vi "Config - access SUM report - REPORT.vi"(5 ".ini Controller":enum16{"Read", "Write"}(ring), 6 "End Time":timestamp, 7 "Start Time":timestamp, 8 "error in":errorcluster, 9 "RVHR Cluster In":T1, 10 "Cluster in":T7 {"Settings Cluster"."Image Frequency" items=["2", "3", "5"]; "Settings Cluster"."Device Resolution" items=["0.1 µm", "1 µm", "10 µm"]; "Settings Cluster"."Distance Format" items=["kilometres", "miles & chains", "metres", "stations", "miles"]; "Settings Cluster"."Sampling Distance" items=["1mm", "2mm"]}, 11 "Config File Ref":T14=refnum) -> (0 "error out":errorcluster, 1 "Dates-Times":T6, 2 "Cluster out":T7 {"Settings Cluster"."Image Frequency" items=["2", "3", "5"]; "Settings Cluster"."Device Resolution" items=["0.1 µm", "1 µm", "10 µm"]; "Settings Cluster"."Distance Format" items=["kilometres", "miles & chains", "metres", "stations", "miles"]; "Settings Cluster"."Sampling Distance" items=["1mm", "2mm"]}, 3 "refnum out":T14)   [LabVIEW 2023]
doc: "This subVI reads/writes initial config data from a .ini file to define the test settings."
uses:
  Controls/File Information CLuster.ctl
  Controls/Run Description.ctl
  Controls/Run information (YRCA).ctl
  Controls/System information (YRCA - Truncate).ctl
  Controls/Sum File Cluster (RCA).ctl
  Controls/Sampling DIstance.ctl
  <vilib>/Utility/config.llb/Config Data RefNum.ctl
  <vilib>/Utility/config.llb/NI_LVConfig.lvlib
  Controls/SUM Cluster.ctl
  Controls/Test Cluster.ctl
  Controls/Distance Units.ctl
  Controls/Settings Cluster.ctl
  Controls/Device_Type.ctl
  Controls/Device_Resolution.ctl
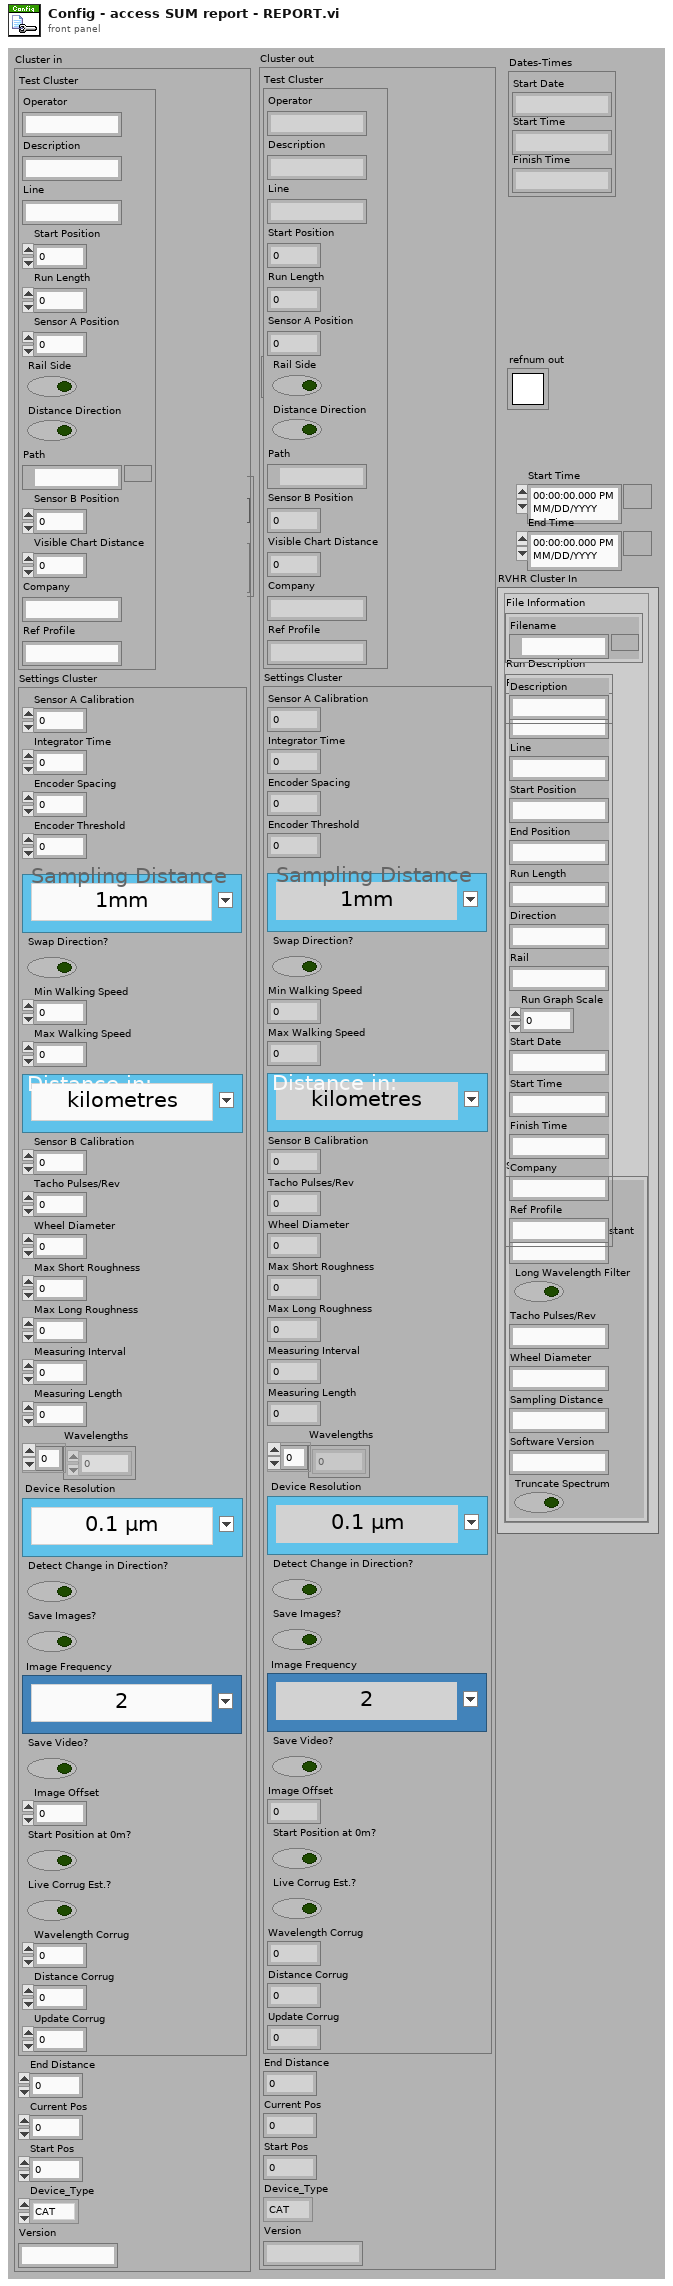
[diagram p1: front panel]
types:
  T1 = typedef "Sum File Cluster (RCA).ctl" = cluster{"File Information":T2, "Run Description":T3, "Run Information":T4, "System Information":T5}
  T2 = typedef "File Information CLuster.ctl" = cluster{"Filename":path}
  T3 = typedef "Run Description.ctl" = cluster{"Description":string}
  T4 = typedef "Run information (YRCA).ctl" = cluster{"Operator":string, "Line":string, "Start Position":string, "End Position":string, "Run Length":string, "Direction":string, "Rail":string, "Run Graph Scale":u16, "Start Date":string, "Start Time":string, "Finish Time":string, "Company":string, "Ref Profile":string}
  T5 = typedef "System information (YRCA - Truncate).ctl" = cluster{"Sensor Calibration":string, "Integrator Time Constant":string, "Long Wavelength Filter":bool, "Tacho Pulses/Rev":string, "Wheel Diameter":string, "Sampling Distance":string, "Software Version":string, "Truncate Spectrum":bool}
  T6 = cluster{"Start Date":string, "Start Time":string, "Finish Time":string}
  T7 = typedef "SUM Cluster.ctl" = cluster{"Test Cluster":T8, "Settings Cluster":T9, "End Distance":dbl, "Current Pos":dbl, "Start Pos":dbl, "Device_Type":T13, "Version":string}
  T8 = typedef "Test Cluster.ctl" = cluster{"Operator":string, "Description":string, "Line":string, "Start Position":dbl, "Run Length":dbl, "Sensor A Position":dbl, "Rail Side":bool, "Distance Direction":bool, "Path":path, "Sensor B Position":dbl, "Visible Chart Distance":dbl, "Company":string, "Ref Profile":string}
  T9 = typedef "Settings Cluster.ctl" = cluster{"Sensor A Calibration":dbl, "Integrator Time":dbl, "Encoder Spacing":dbl, "Encoder Threshold":dbl, "Sampling Distance":T10, "Swap Direction?":bool, "Min Walking Speed":dbl, "Max Walking Speed":dbl, "Distance Format":T11, "Sensor B Calibration":dbl, "Tacho Pulses/Rev":dbl, "Wheel Diameter":dbl, "Max Short Roughness":dbl, "Max Long Roughness":dbl, "Measuring Interval":dbl, "Measuring Length":dbl, "Wavelengths":dbl[], "Device Resolution":T12, "Detect Change in Direction?":bool, "Save Images?":bool, "Image Frequency":T10, "Save Video?":bool, "Image Offset":dbl, "Start Position at 0m?":bool, "Live Corrug Est.?":bool, "Wavelength Corrug":u8, "Distance Corrug":u8, "Update Corrug":u8}
  T10 = typedef "Sampling DIstance.ctl" = u16
  T11 = typedef "Distance Units.ctl" = u16
  T12 = typedef "Device_Resolution.ctl" = u16
  T13 = typedef "Device_Type.ctl" = enum16{"CAT", "Bi-CAT", "YRCA", "RCA", "RV-HR", "TV-HR"}
  T14 = typedef "NI_LVConfig.lvlib/Config Data RefNum.ctl" = refnum<k1>
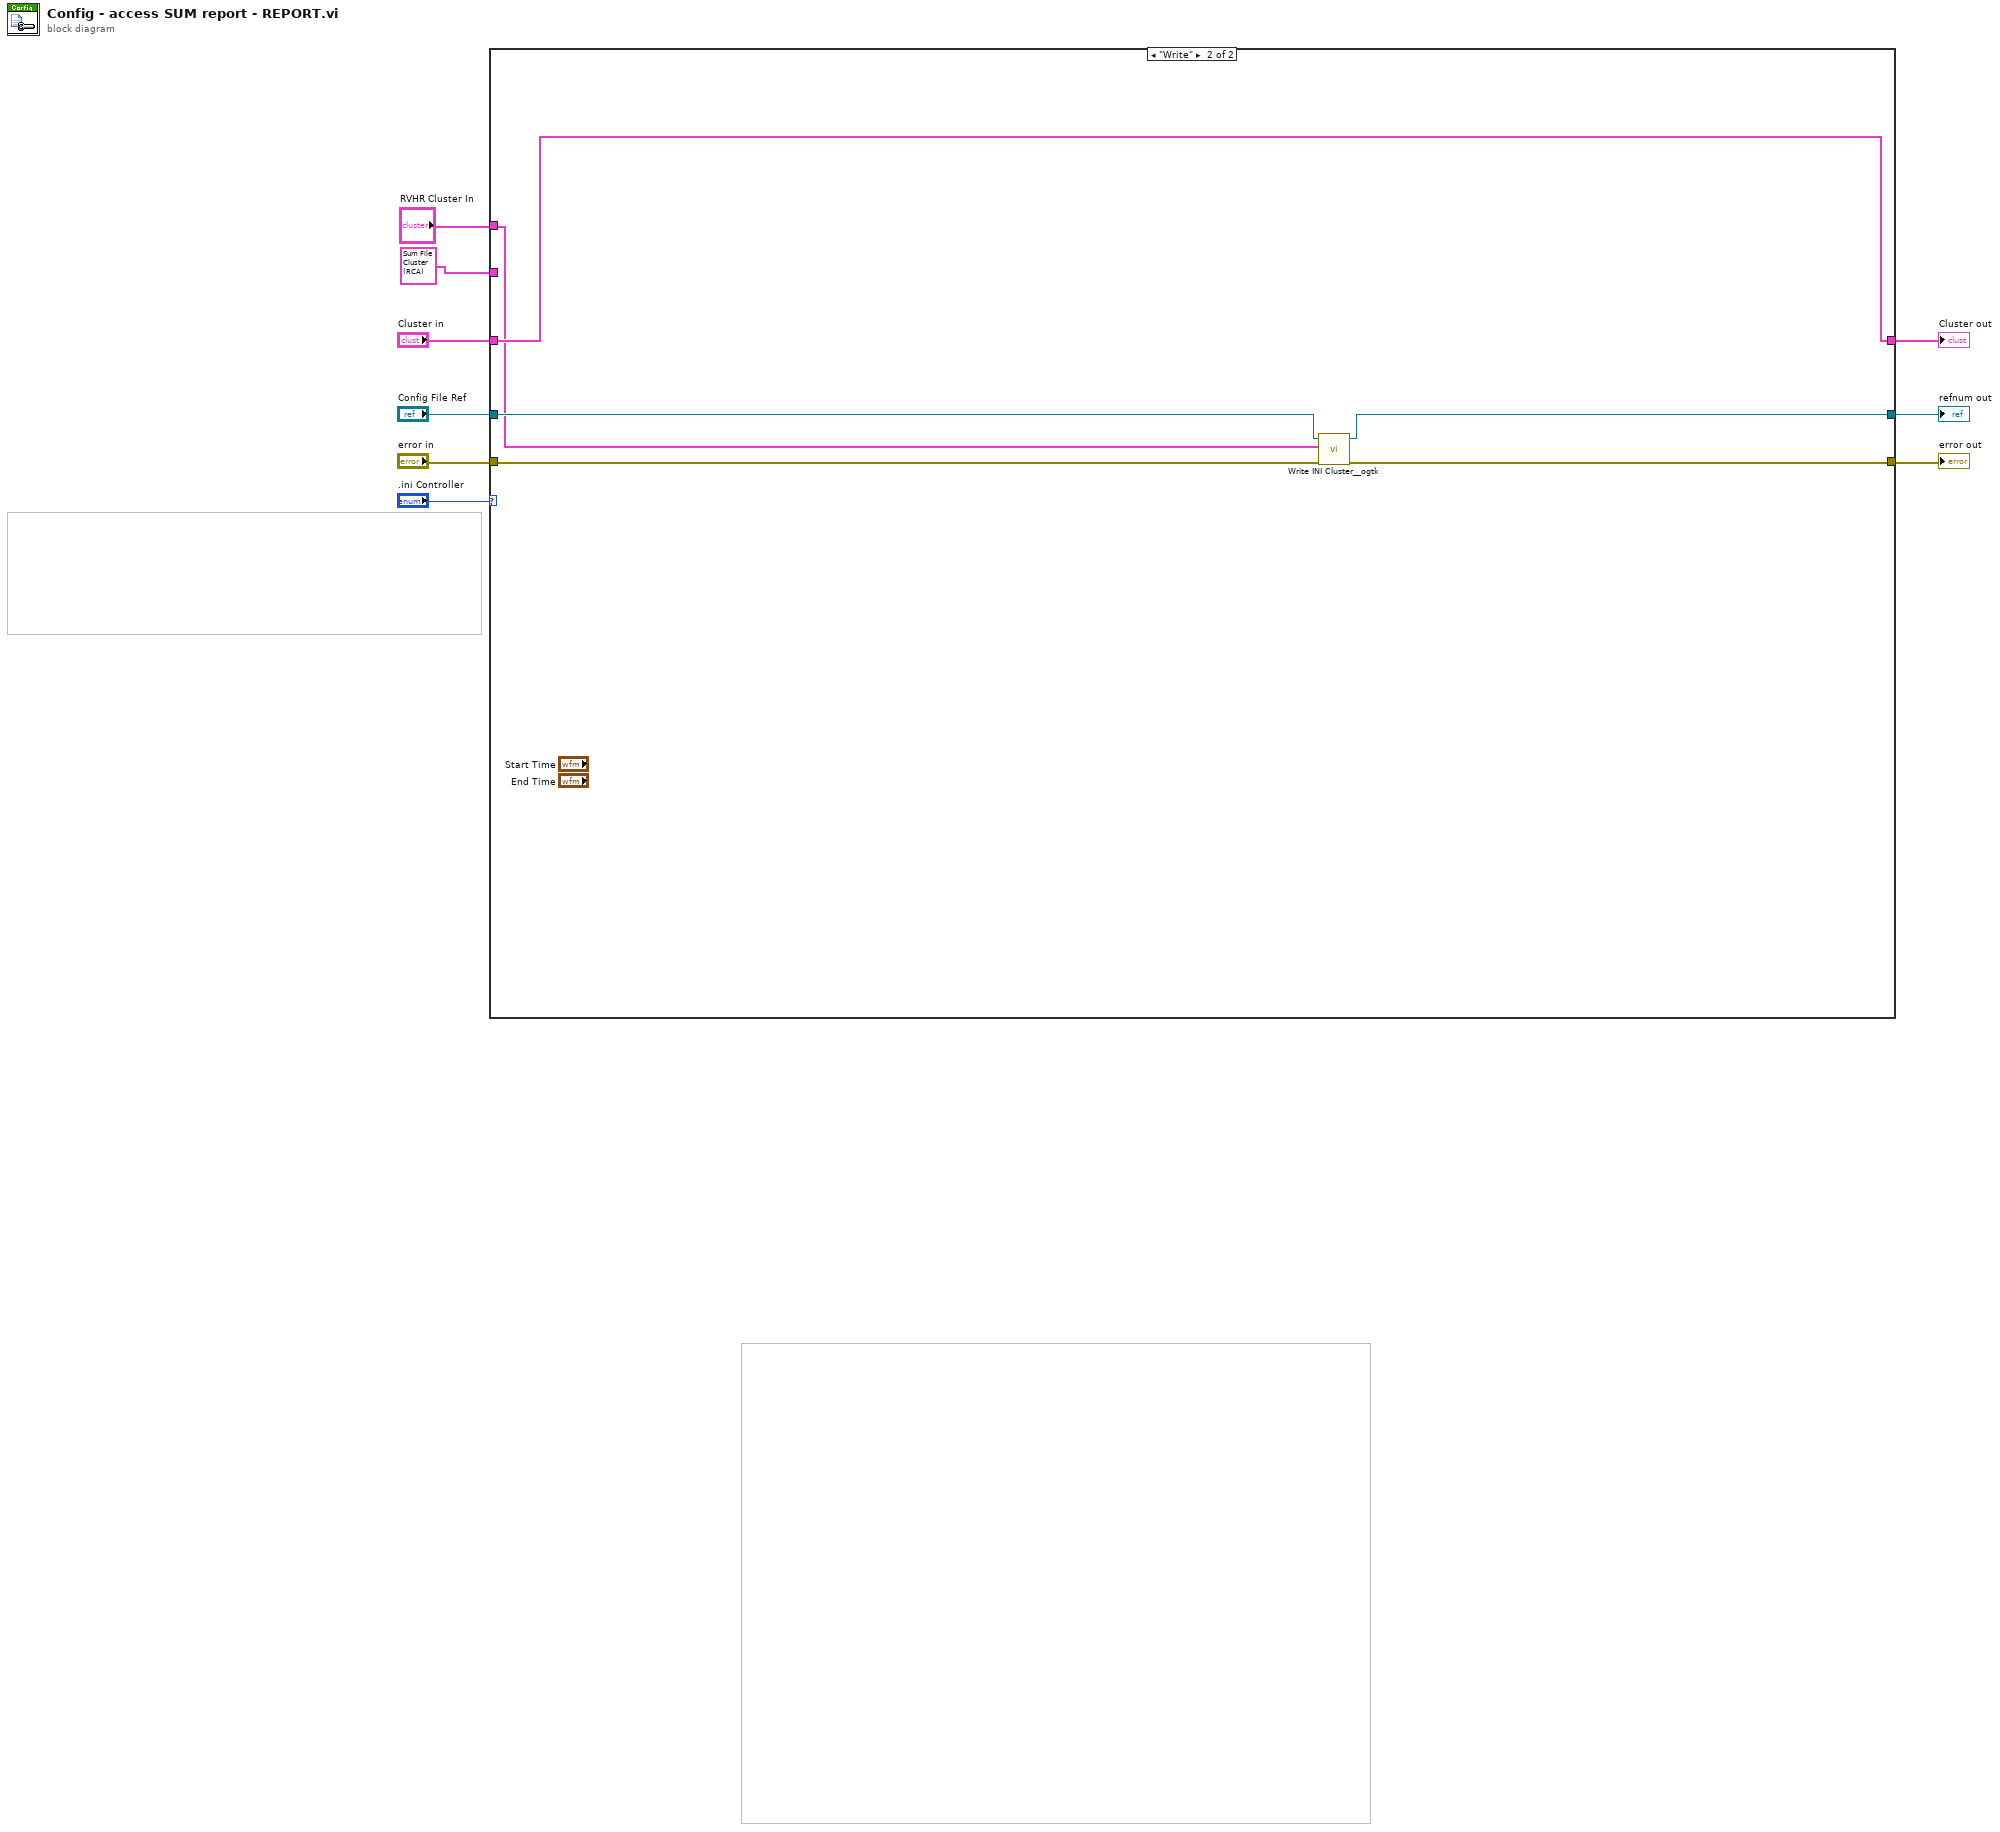
[diagram p0: block diagram]
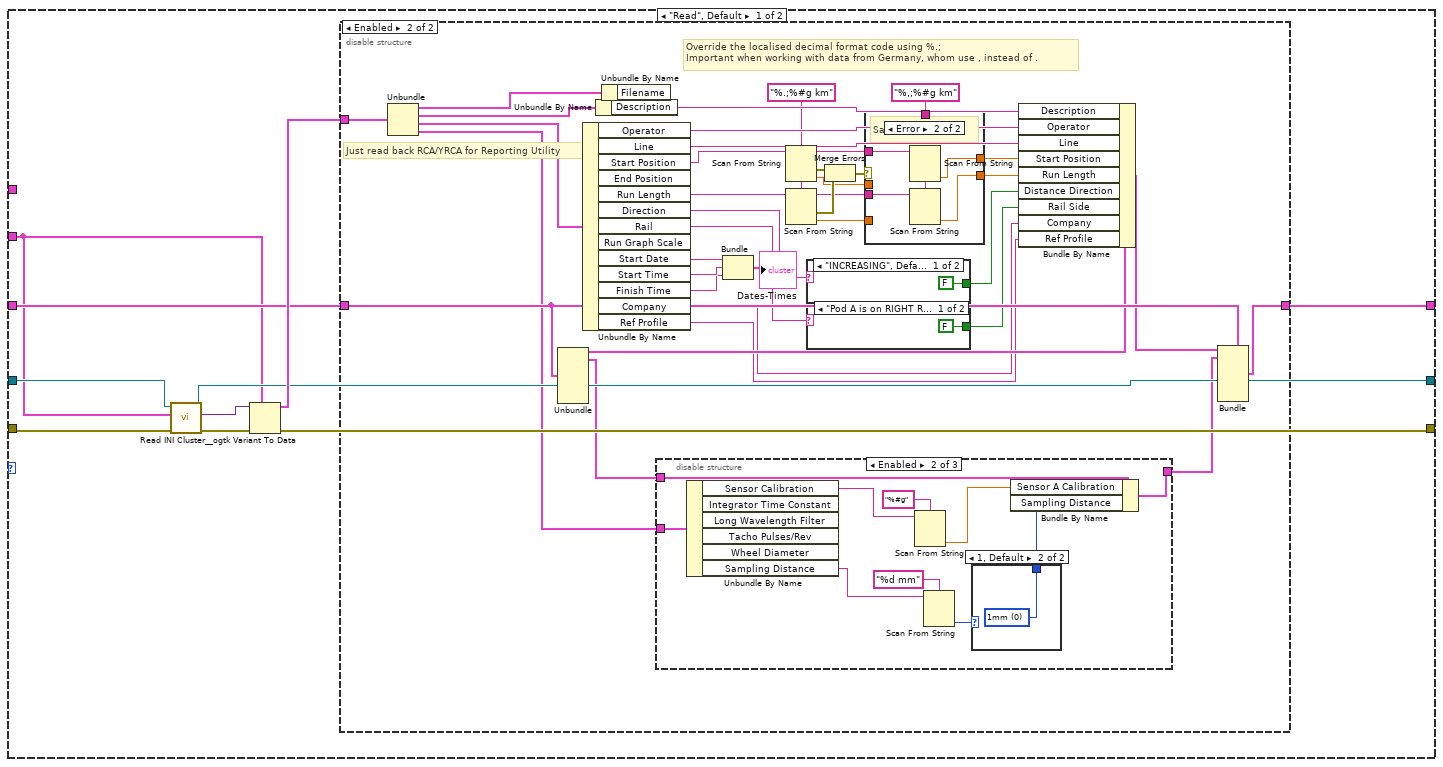
[diagram p2: hidden frame]
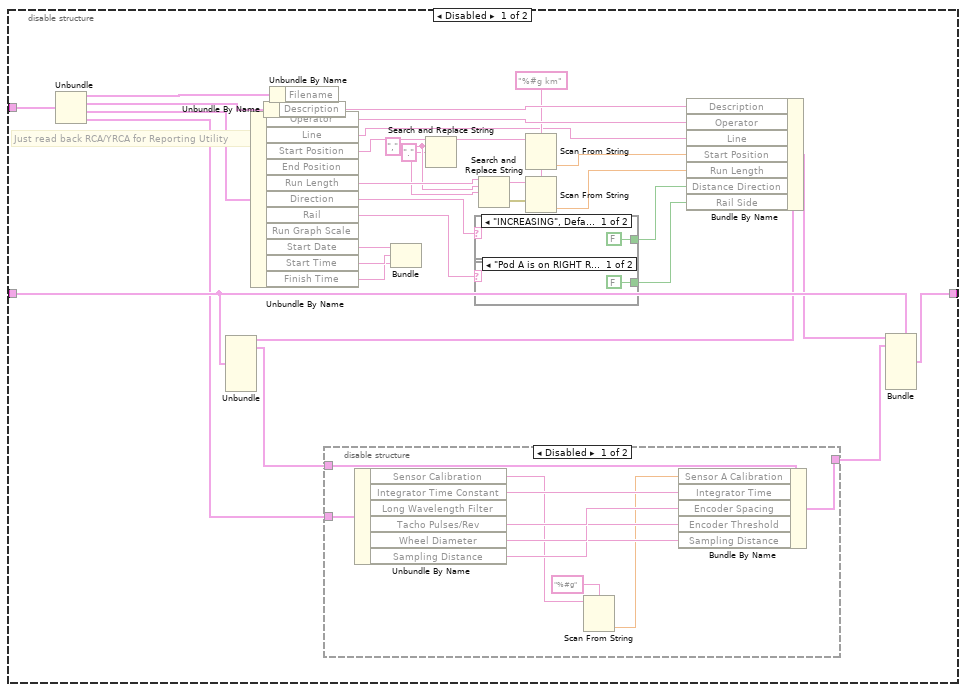
[diagram p3: hidden frame]
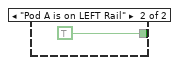
[diagram p4: hidden frame]
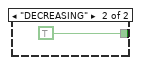
[diagram p5: hidden frame]
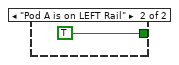
[diagram p8: hidden frame]
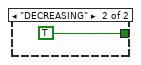
[diagram p9: hidden frame]
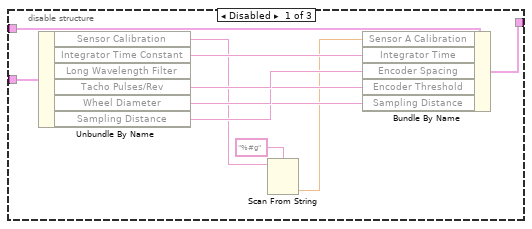
[diagram p10: hidden frame]
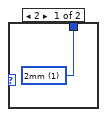
[diagram p11: hidden frame]
diagram:
  n1 = case shown="\"Write\"" ".ini Controller" {
    tunnel: [w19 w137] -> w8
    tunnel: "Config File Ref" -> [w16 w136]
    tunnel: [w11 w135] -> w7
    tunnel: "Cluster in" -> [w12 w134]
    tunnel: [w13 w134] -> w3
    tunnel: "error in" -> [w17 w138]
    tunnel: T1 {"File Information"={"Filename"=path ""}, "Run Description"={"Description"=""}, "Run Information"={"Operator"="", "Line"="", "Start Position"="", "End Position"="", "Run Length"="", "Direction"="", "Rail"="", "Run Graph Scale"=0, "Start Date"="", "Start Time"="", "Finish Time"="", "Company"="", "Ref Profile"=""}, "System Information"={"Sensor Calibration"="", "Integrator Time Constant"="", "Long Wavelength Filter"=FALSE, "Tacho Pulses/Rev"="", "Wheel Diameter"="", "Sampling Distance"="", "Software Version"="", "Truncate Spectrum"=FALSE}} ("output cluster") -> [w10 _]
    tunnel: "RVHR Cluster In" -> [_ w133]
    frame "Read", Default {
      n2 = call "Read INI Cluster__ogtk.vi"("error in (no error)"=w17, "INI Fomatted Cluster Type"=w10, "refnum"=w16) -> ("error out"=w18:errorcluster, "INI Fomatted Cluster"=w15:variant, "dup refnum"=w11:T14)  [unwired: 4 in, 2 out]
      n3 = Variant To Data(error in=w18, type=w10, Variant=w15) -> (data=w14:T1, error out=w19:errorcluster)
      n4 = disable-structure shown="Enabled" {
        disable-tunnel: w14 -> [w50 w99]
        disable-tunnel: [w49 w98] -> w13
        disable-tunnel: w12 -> [w48 w97]
        frame Disabled {
          w20 = "." ("replace string (\"\")")
          w21 = "," ("search string")
          w36 = "%#g km" ("format string")
          # "Just read back RCA/YRCA for Reporting Utility"
          n5 = Unbundle(w50) -> ("File Information"=w43:T2, "Run Description"=w46:T3, "Run Information"=w45:T4, "System Information"=w39:T5)
          n6 = Unbundle(w48) -> ("Test Cluster"=w47:T8, "Settings Cluster"=w41:T9)  [unwired: 5 out]
          n7 = Unbundle By Name(w45) -> ("Operator"=w44:string, "Line"=w27:string, "Start Position"=w26:string, "Run Length"=w22:string, "Direction"=w34:string, "Rail"=w32:string, "Start Date"=w30:string, "Start Time"=w29:string, "Finish Time"=w28:string)  [unwired: 2 out]
          n8 = Unbundle By Name(w46) -> ("Description"=w38:string)
          n9 = Unbundle By Name(w43) -> ()  [unwired: 1 out]
          n10 = disable-structure shown="Disabled" {
            disable-tunnel: w41 -> [w64 _]
            disable-tunnel: [w63 _] -> w40
            disable-tunnel: w39 -> [w62 _]
            frame Disabled {
              n11 = Unbundle By Name(w62) -> ("Sensor Calibration"=w57:string, "Integrator Time Constant"=w61:string, "Tacho Pulses/Rev"=w60:string, "Wheel Diameter"=w59:string, "Sampling Distance"=w58:string)  [unwired: 1 out]
              n12 = Scan From String(format string="%#g", input string=w57) -> (output 1=w55:dbl)  [unwired: 3 in, 3 out]
              n13 = Bundle By Name(cluster=w64, "Sensor A Calibration"=w55, "Integrator Time"=w61, "Encoder Spacing"=w60, "Encoder Threshold"=w59, "Sampling Distance"=w58) -> (w63:T9)
            }
            frame Enabled {
            }
          }
          n14 = Bundle("Start Date"=w30, "Start Time"=w29, "Finish Time"=w28) -> ()  [unwired: 1 in, 1 out]
          n15 = Search and Replace String(input string=w26, search string=w21, replace string=w20) -> (result string=w25:string)  [unwired: 5 in, 3 out]
          n16 = case shown="\"INCREASING\", Default" w34 {
            tunnel: [FALSE ("Distance Direction") TRUE ("Distance Direction")] -> w33
            frame "INCREASING", Default {
            }
            frame "DECREASING" {
            }
          }
          n17 = case shown="\"Pod A is on RIGHT Rail\", Default" w32 {
            tunnel: [FALSE ("Distance Direction") TRUE ("Distance Direction")] -> w31
            frame "Pod A is on RIGHT Rail", Default {
            }
            frame "Pod A is on LEFT Rail" {
            }
          }
          n18 = Search and Replace String(input string=w22, search string=w21, replace string=w20) -> (result string=w24:string, error out=w23:errorcluster)  [unwired: 5 in, 2 out]
          n19 = Scan From String(format string=w36, input string=w25) -> (output 1=w37:dbl)  [unwired: 3 in, 3 out]
          n20 = Scan From String(format string=w36, input string=w24, error in=w23) -> (output 1=w35:dbl)  [unwired: 2 in, 3 out]
          n21 = Bundle By Name(cluster=w47, "Description"=w38, "Operator"=w44, "Line"=w27, "Start Position"=w37, "Run Length"=w35, "Distance Direction"=w33, "Rail Side"=w31) -> (w42:T8)
          n22 = Bundle(cluster=w48, "Test Cluster"=w42, "Settings Cluster"=w40) -> (w49:T7)  [unwired: 5 in]
        }
        frame Enabled {
          w86 = "%.;%#g km" ("format string")
          # "Override the localised decimal format code using %.;\nImportant when working with data from Germany, whom use , instead of ."
          # "Just read back RCA/YRCA for Reporting Utility"
          n23 = Unbundle(w99) -> ("File Information"=w92:T2, "Run Description"=w95:T3, "Run Information"=w94:T4, "System Information"=w88:T5)
          n24 = Unbundle(w97) -> ("Test Cluster"=w96:T8, "Settings Cluster"=w90:T9)  [unwired: 5 out]
          n25 = Unbundle By Name(w94) -> ("Operator"=w93:string, "Line"=w78:string, "Start Position"=w72:string, "Run Length"=w71:string, "Direction"=w85:string, "Rail"=w83:string, "Start Date"=w81:string, "Start Time"=w80:string, "Finish Time"=w79:string, "Company"=w66:string, "Ref Profile"=w65:string)  [unwired: 2 out]
          n26 = Unbundle By Name(w95) -> ("Description"=w87:string)
          n27 = Unbundle By Name(w92) -> ()  [unwired: 1 out]
          n28 = disable-structure shown="Enabled" {
            disable-tunnel: w90 -> [w120 w130 _]
            disable-tunnel: [w119 w129 _] -> w89
            disable-tunnel: w88 -> [w118 w128 _]
            frame Disabled {
              n29 = Unbundle By Name(w118) -> ("Sensor Calibration"=w113:string, "Integrator Time Constant"=w117:string, "Tacho Pulses/Rev"=w116:string, "Wheel Diameter"=w115:string, "Sampling Distance"=w114:string)  [unwired: 1 out]
              n30 = Scan From String(format string="%#g", input string=w113) -> (output 1=w111:dbl)  [unwired: 3 in, 3 out]
              n31 = Bundle By Name(cluster=w120, "Sensor A Calibration"=w111, "Integrator Time"=w117, "Encoder Spacing"=w116, "Encoder Threshold"=w115, "Sampling Distance"=w114) -> (w119:T9)
            }
            frame Enabled {
              n32 = Unbundle By Name(w128) -> ("Sensor Calibration"=w127:string, "Sampling Distance"=w123:string)  [unwired: 4 out]
              n33 = Scan From String(format string="%#g", input string=w127) -> (output 1=w125:dbl)  [unwired: 3 in, 3 out]
              n34 = Scan From String(format string="%d mm", input string=w123) -> (output 1=w121:i32)  [unwired: 3 in, 3 out]
              n35 = case shown="1, Default" w121 {
                tunnel: [w131 w132] -> w122
                frame 2 {
                  w131 = T10 1 items=["1mm", "2mm"] ("Sampling Distance")
                }
                frame 1, Default {
                  w132 = T10 0 items=["1mm", "2mm"] ("Sampling Distance")
                }
              }
              n36 = Bundle By Name(cluster=w130, "Sensor A Calibration"=w125, "Sampling Distance"=w122) -> (w129:T9)
            }
            frame Disabled {
            }
          }
          n37 = Bundle("Start Date"=w81, "Start Time"=w80, "Finish Time"=w79) -> (→"Dates-Times":T6)  [unwired: 1 in]
          n38 = Scan From String(format string=w86, input string=w72) -> (error out=w76:errorcluster, output 1=w67:dbl)  [unwired: 3 in, 2 out]
          n39 = Scan From String(format string=w86, input string=w71) -> (error out=w74:errorcluster, output 1=w68:dbl)  [unwired: 3 in, 2 out]
          n40 = case shown="\"INCREASING\", Default" w85 {
            tunnel: [FALSE ("Distance Direction") TRUE ("Distance Direction")] -> w84
            frame "INCREASING", Default {
            }
            frame "DECREASING" {
            }
          }
          n41 = case shown="\"Pod A is on RIGHT Rail\", Default" w83 {
            tunnel: [FALSE ("Distance Direction") TRUE ("Distance Direction")] -> w82
            frame "Pod A is on RIGHT Rail", Default {
            }
            frame "Pod A is on LEFT Rail" {
            }
          }
          n42 = Merge Errors(w76, w74) -> (w75:errorcluster)
          n43 = case shown="Error" w75 {
            tunnel: "%,;%#g km" ("format string") -> [_ w106]
            tunnel: w72 -> [_ w105]
            tunnel: w71 -> [_ w104]
            tunnel: [w100 w103] -> w70
            tunnel: [w101 w102] -> w69
            tunnel: w68 -> [w101 _]
            tunnel: w67 -> [w100 _]
            frame No Error {
            }
            frame Error {
              # "Saved with comma"
              n44 = Scan From String(format string=w106, input string=w105) -> (output 1=w103:dbl)  [unwired: 3 in, 3 out]
              n45 = Scan From String(format string=w106, input string=w104) -> (output 1=w102:dbl)  [unwired: 3 in, 3 out]
            }
          }
          n46 = Bundle By Name(cluster=w96, "Description"=w87, "Operator"=w93, "Line"=w78, "Start Position"=w70, "Run Length"=w69, "Distance Direction"=w84, "Rail Side"=w82, "Company"=w66, "Ref Profile"=w65) -> (w91:T8)
          n47 = Bundle(cluster=w97, "Test Cluster"=w91, "Settings Cluster"=w89) -> (w98:T7)  [unwired: 5 in]
        }
      }
    }
    frame "Write" {
      n48 = call "Write INI Cluster__ogtk.vi"("error in (no error)"=w138, "INI Fomatted Cluster"=w133, "refnum"=w136) -> ("error out"=w137:errorcluster, "dup refnum"=w135:T14)  [unwired: 7 in]
    }
  }
  "error out" <- w8
  "refnum out" <- w7
  "Cluster out" <- w3
